vi "Initialization VI.vi"(8 "error in (no error)":errorcluster, 10 "Custom XML":string, 11 "Device Item Ref in":T1 format="%.0x") -> (0 "error out":errorcluster, 3 "Device Item Ref out":T1 format="%.0x")   [LabVIEW 2019, in "TimingDRV System Explorer.lvlib"]
uses:
  TimingDRV System Explorer.lvlib
  <vilib>/NI VeriStand/Custom Device API/Custom Device Item Ref.ctl
  Engine/Parent Classes/Process/Process.lvclass
  Engine/Processes/Single Stepped TS/STS Process.lvclass
  C:/Users/nitest/Desktop/CD Project Tools/Source/Engine/Parent Classes/Process/Process.lvclass
  Engine/Processes/TCP Process/TCP Process.lvclass
  Engine/Processes/Free Running TS/FRTS Process.lvclass
  <vilib>/NI VeriStand/Custom Device API/Set Item Property (String).vi
  <vilib>/NI VeriStand/Custom Device API/Set Item Property (I32).vi
  <vilib>/NI VeriStand/Custom Device API/Custom Device API.lvlib
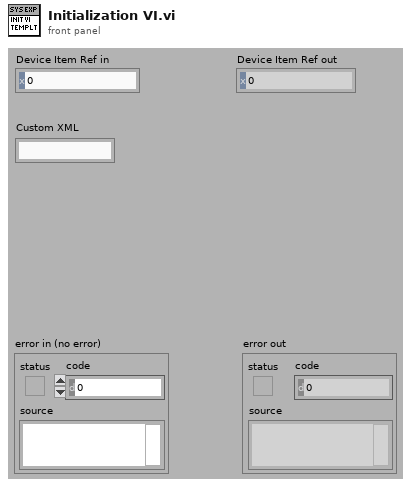
[diagram p1: front panel]
types:
  T1 = typedef "Custom Device API.lvlib/Custom Device Item Ref.ctl" = u64
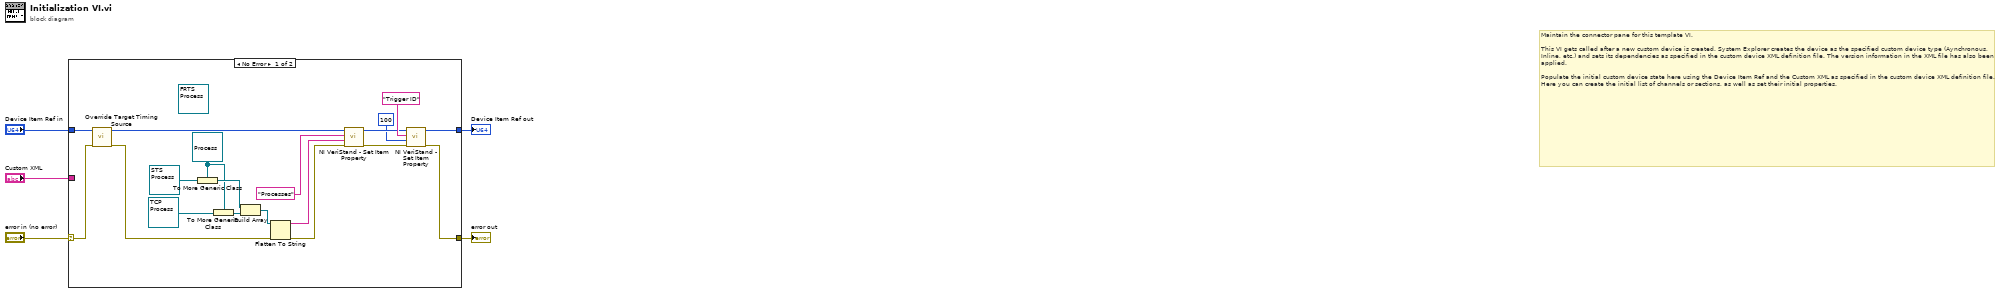
[diagram p0: block diagram]
diagram:
  # "Maintain the connector pane for this template VI.\n\nThis VI gets called after a new custom device is created. System Explorer creates the device as the specified custom device type (Aynchronous, Inline, etc.) and sets its dependencies as specified in the custom device XML definition file. The version information in the XML file has also been applied.\n\nPopulate the initial custom device state here using the Device Item Ref and the Custom XML as specified in the custom device XML definition file. Here you can create the initial list of channels or sections, as well as set their initial properties."
  n1 = case shown="No Error" "error in (no error)" {
    selector: "error in (no error)" -> [w12 w26]
    tunnel: [w17 w26] -> w5
    tunnel: [w18 w25] -> w3
    tunnel: "Device Item Ref in" -> [w13 w25]
    tunnel: "Custom XML" -> [_ _]
    frame No Error {
      (unwired) refnum<class "FRTS Process.lvclass"> refnum ("TimingDRV Engine.lvlib:FRTS Process.lvclass")
      w7 = refnum<class "Process.lvclass"> refnum ("TelemetryAsync Engine.lvlib:Process.lvclass")
      n2 = call "Override Target Timing Source.vi"("error in (no error)"=w12, "CD Ref in"=w13) -> ("error out"=w14:errorcluster, "CD Ref out"=w15:T1)  [unwired: 8 in]
      n3 = To More Generic Class(target class=w7, reference=refnum<class "STS Process.lvclass"> refnum ("TimingDRV Engine.lvlib:STS Process.lvclass")) -> (generic class reference=w10:refnum<class "Process.lvclass">)
      n4 = To More Generic Class(target class=w7, reference=refnum<class "TCP Process.lvclass"> refnum ("TimingDRV Engine.lvlib:TCP Process.lvclass")) -> (generic class reference=w6:refnum<class "Process.lvclass">)
      n5 = Build Array(w10, w6) -> (w9:refnum<class "Process.lvclass">[])
      n6 = Flatten To String(anything=w9, error in (no error)=w14) -> (data string=w23:string, error out=w22:errorcluster)  [unwired: 2 in, 1 out]
      n7 = call-poly <vilib>:"NI VeriStand - Set Item Property.vi"("error in (no error)"=w22, "Value"=w23, "Property Name"="Processes", "Item Ref in"=w15) -> ("error out"=w19:errorcluster, "Item Ref out"=w20:T1)  [unwired: 5 in, 1 out]
      n8 = call-poly <vilib>:"NI VeriStand - Set Item Property.vi"("error in (no error)"=w19, "Value"=100, "Property Name"="Trigger ID", "Item Ref in"=w20) -> ("error out"=w17:errorcluster, "Item Ref out"=w18:T1)  [unwired: 5 in, 1 out]
    }
    frame Error {
    }
  }
  "error out" <- w5
  "Device Item Ref out" <- w3
